vi "IO.vi"(8 "error in":errorcluster) -> (0 "error out":errorcluster, 3 "task out":refnum<k21>)   [LabVIEW 2011]
uses:
  <vilib>/DAQmx/create/channels.llb/DAQmx Create Channel (AO-Voltage-Basic).vi
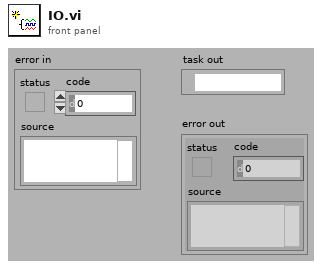
[diagram p1: front panel]
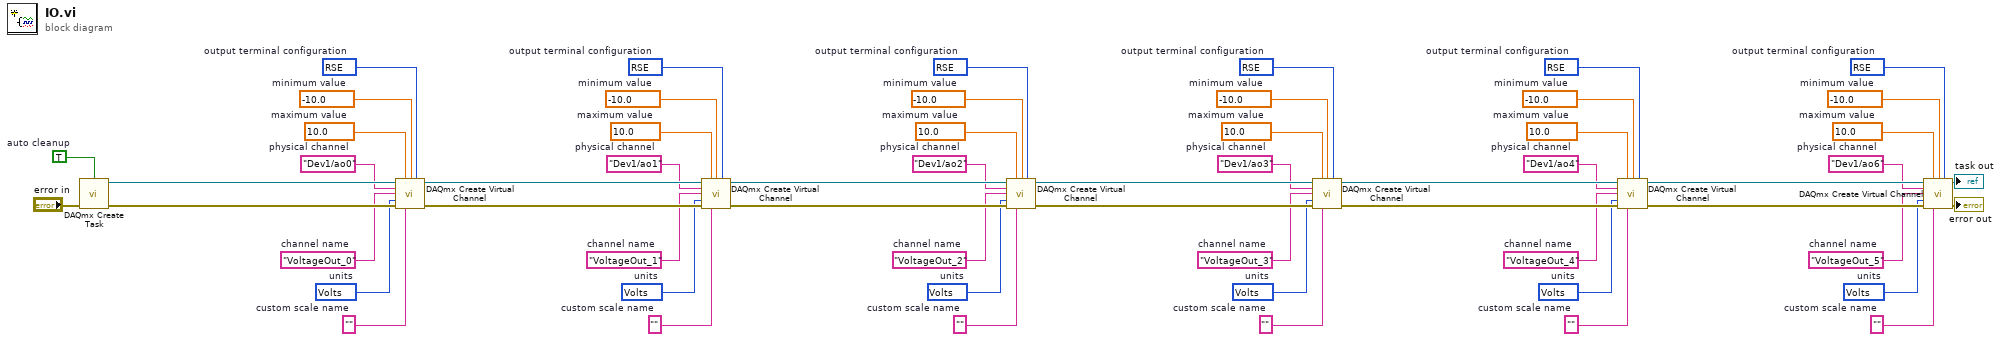
[diagram p0: block diagram]
diagram:
  w1 = 10083 items=["Default"=-1, "RSE"=10083, "Differential"=10106, "Pseudodifferential"=12529]  # output terminal configuration
  w2 = 10348 items=["Volts"=10348, "From Custom Scale"=10065]  # units
  w3 = "VoltageOut_5"  # channel name
  w6 = ""  # custom scale name
  w7 = -10.0  # minimum value
  w8 = 10.0  # maximum value
  w9 = "Dev1/ao6"  # physical channel
  w11 = 10083 items=["Default"=-1, "RSE"=10083, "Differential"=10106, "Pseudodifferential"=12529]  # output terminal configuration
  w12 = 10348 items=["Volts"=10348, "From Custom Scale"=10065]  # units
  w13 = "VoltageOut_4"  # channel name
  w15 = ""  # custom scale name
  w16 = -10.0  # minimum value
  w17 = 10.0  # maximum value
  w18 = "Dev1/ao4"  # physical channel
  w20 = 10083 items=["Default"=-1, "RSE"=10083, "Differential"=10106, "Pseudodifferential"=12529]  # output terminal configuration
  w21 = 10348 items=["Volts"=10348, "From Custom Scale"=10065]  # units
  w22 = "VoltageOut_3"  # channel name
  w24 = ""  # custom scale name
  w25 = -10.0  # minimum value
  w26 = 10.0  # maximum value
  w27 = "Dev1/ao3"  # physical channel
  w29 = 10083 items=["Default"=-1, "RSE"=10083, "Differential"=10106, "Pseudodifferential"=12529]  # output terminal configuration
  w30 = 10348 items=["Volts"=10348, "From Custom Scale"=10065]  # units
  w31 = "VoltageOut_2"  # channel name
  w33 = ""  # custom scale name
  w34 = -10.0  # minimum value
  w35 = 10.0  # maximum value
  w36 = "Dev1/ao2"  # physical channel
  w38 = 10083 items=["Default"=-1, "RSE"=10083, "Differential"=10106, "Pseudodifferential"=12529]  # output terminal configuration
  w39 = 10348 items=["Volts"=10348, "From Custom Scale"=10065]  # units
  w40 = "VoltageOut_1"  # channel name
  w42 = ""  # custom scale name
  w43 = -10.0  # minimum value
  w44 = 10.0  # maximum value
  w45 = "Dev1/ao1"  # physical channel
  w47 = 10083 items=["Default"=-1, "RSE"=10083, "Differential"=10106, "Pseudodifferential"=12529]  # output terminal configuration
  w48 = 10348 items=["Volts"=10348, "From Custom Scale"=10065]  # units
  w49 = "VoltageOut_0"  # channel name
  w51 = ""  # custom scale name
  w52 = -10.0  # minimum value
  w53 = 10.0  # maximum value
  w54 = "Dev1/ao0"  # physical channel
  w56 = TRUE  # auto cleanup
  n1 = call <vilib>:"DAQmx Create Task.vi"("auto cleanup"=w56, "error in"="error in") -> ("task out"=w55:refnum<k21>, "error out"=w57:errorcluster)  [unwired: 3 in, 9 out]
  n2 = call-poly <vilib>:"DAQmx Create Virtual Channel.vi"("task in"=w55, "maximum value"=w53, "minimum value"=w52, "output terminal configuration"=w47, "physical channels"=w54, "name to assign"=w49, "units"=w48, "error in"=w57, "custom scale name"=w51) -> ("task out"=w46:refnum<k21>, "error out"=w50:errorcluster)  [unwired: 1 in, 4 out]
  n3 = call-poly <vilib>:"DAQmx Create Virtual Channel.vi"("task in"=w46, "maximum value"=w44, "minimum value"=w43, "output terminal configuration"=w38, "physical channels"=w45, "name to assign"=w40, "units"=w39, "error in"=w50, "custom scale name"=w42) -> ("task out"=w37:refnum<k21>, "error out"=w41:errorcluster)  [unwired: 1 in, 4 out]
  n4 = call-poly <vilib>:"DAQmx Create Virtual Channel.vi"("task in"=w37, "maximum value"=w35, "minimum value"=w34, "output terminal configuration"=w29, "physical channels"=w36, "name to assign"=w31, "units"=w30, "error in"=w41, "custom scale name"=w33) -> ("task out"=w28:refnum<k21>, "error out"=w32:errorcluster)  [unwired: 1 in, 4 out]
  n5 = call-poly <vilib>:"DAQmx Create Virtual Channel.vi"("task in"=w28, "maximum value"=w26, "minimum value"=w25, "output terminal configuration"=w20, "physical channels"=w27, "name to assign"=w22, "units"=w21, "error in"=w32, "custom scale name"=w24) -> ("task out"=w19:refnum<k21>, "error out"=w23:errorcluster)  [unwired: 1 in, 4 out]
  n6 = call-poly <vilib>:"DAQmx Create Virtual Channel.vi"("task in"=w19, "maximum value"=w17, "minimum value"=w16, "output terminal configuration"=w11, "physical channels"=w18, "name to assign"=w13, "units"=w12, "error in"=w23, "custom scale name"=w15) -> ("task out"=w10:refnum<k21>, "error out"=w14:errorcluster)  [unwired: 1 in, 4 out]
  n7 = call-poly <vilib>:"DAQmx Create Virtual Channel.vi"("task in"=w10, "maximum value"=w8, "minimum value"=w7, "output terminal configuration"=w1, "physical channels"=w9, "name to assign"=w3, "units"=w2, "error in"=w14, "custom scale name"=w6) -> ("task out"=→"task out":refnum<k21>, "error out"=→"error out":errorcluster)  [unwired: 1 in, 4 out]
